vi "Channel ID to Tree Items.vi"(8 "error in (no error)":errorcluster, 9 "Channel ID":string, 10 "Indent":i32, 11 "Refnum in":T1) -> (0 "error out":errorcluster, 2 "Items":T2(array[cluster]), 3 "Refnum out":T1)   [LabVIEW 2017]
uses:
  DSF Configuration API/1.0.0/Public/Controls/DSF Config Data RefNum.ctl
  Tree Item Type.ctl
  DSF Configuration API/1.0.0/Public/Read Item/Read Channel.vi
  DSF Configuration API/1.0.0/Public/Read Item/Read Settings.vi
  DSF Configuration API/1.0.0/DSF Configuration API.lvlib
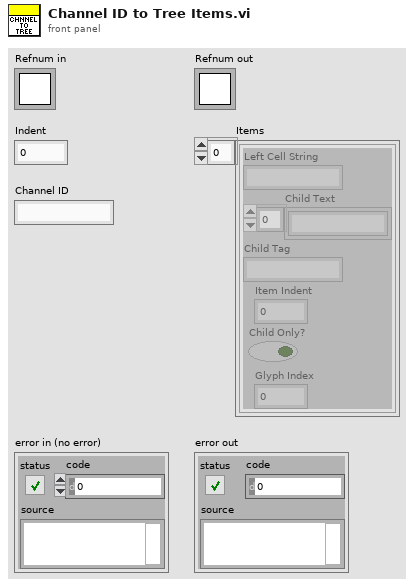
[diagram p1: front panel]
types:
  T1 = typedef "DSF Configuration API.lvlib/DSF Config Data RefNum.ctl" = refnum<k1>
  T2 = cluster{"Left Cell String":string, "Child Text":string[], "Child Tag":string, "Item Indent":i32, "Child Only?":bool, "Glyph Index":i32}[]
  T3 = typedef "Tree Item Type.ctl" = enum16{"Plugin", "Group", "Transfer", "Channel", "Setting"}
  T4 = typedef "DSF Configuration API.lvlib/DSF Channel Info.ctl" = cluster{"count":i32, "offset":i32, "data type":i32, "resource path":string, "settings id":string}
  T5 = cluster{"Left Cell String":string, "Child Text":string[], "Child Tag":string, "Item Indent":i32, "Child Only?":bool, "Glyph Index":i32}
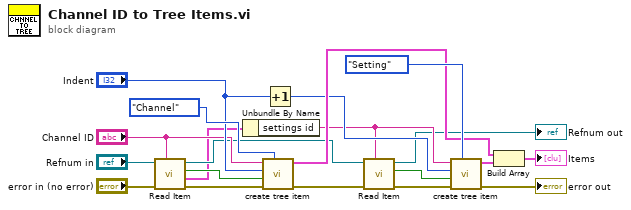
[diagram p0: block diagram]
diagram:
  n1 = call-poly "Read Item.vi"("name"="Channel ID", "error in (no error)"="error in (no error)", "refnum"="Refnum in") -> ("error out"=w15:errorcluster, "value"=w2:T4, "found?"=w7:bool, "refnum out"=w3:T1)  [unwired: 5 in]
  n2 = Unbundle By Name(w2) -> ("settings id"=w9:string)
  n3 = call "create tree item.vi"("Item Type"=Tree_Item_Type."Channel", "error in"=w15, "found?"=w7, "Indent"="Indent", "Left Cell String"="Channel ID") -> ("error out"=w16:errorcluster, "Item"=w12:T5)  [unwired: 5 in]
  n4 = Increment(x="Indent") -> (x+1=w10:i32)
  n5 = call-poly "Read Item.vi"("name"=w9, "error in (no error)"=w16, "refnum"=w3) -> ("error out"=w17:errorcluster, "found?"=w11:bool, "refnum out"=→"Refnum out":T1)  [unwired: 5 in, 1 out]
  n6 = call "create tree item.vi"("Item Type"=Tree_Item_Type."Setting", "error in"=w17, "found?"=w11, "Indent"=w10, "Left Cell String"=w9) -> ("error out"=→"error out":errorcluster, "Item"=w13:T5)  [unwired: 5 in]
  n7 = Build Array(w12, w13) -> (→"Items":T2)
